vi "Render Non-Empty List Section.vi"(8 "Error In":errorcluster) -> (0 "Error Out":errorcluster)   [LabVIEW 2018, in "Tests.lvlib" / "Render.lvlib"]
uses:
  Render.lvlib
  <vilib>/addons/_JKI Toolkits/Caraya/classes/Test/Test.lvclass
  <vilib>/addons/_JKI Toolkits/Caraya/classes/Assert/Assert.lvclass
  src/Toolkit/Toolkit.lvlib
  src/Toolkit/Data/Map/Map.lvclass
  src/Toolkit/Data/Array/Array.lvclass
  src/Toolkit/Low-Level/Support/Lex String.vi
  src/Toolkit/Data/Map/Support/From Datum.vi
  src/Toolkit/Low-Level/Support/Render to String.vi
  src/Toolkit/Data/Array/Support/From Mapped Strings.vi
  src/Toolkit/Low-Level/Context/Compiler.lvclass
  D:/Users/cfield/Code/Field R&D Services/Labstache/src/Toolkit/Data/Datum/Datum.lvclass
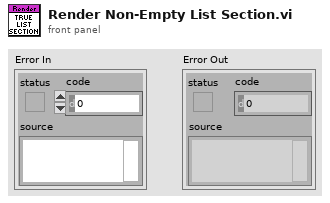
[diagram p1: front panel]
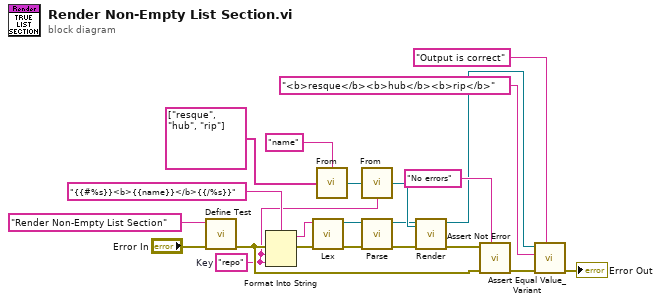
[diagram p0: block diagram]
diagram:
  w4 = "repo"  # Key
  n1 = call <vilib>:"Define Test.vi"("error in (no error)"="Error In", "Label (VI Title)"="Render Non-Empty List Section") -> ("error out"=w10:errorcluster)  [unwired: 9 in]
  n2 = Format Into String(format string="{{#%s}}<b>{{name}}</b>{{/%s}}", error in=w10, w4, w4) -> (resulting string=w7:string, error out=w9:errorcluster)  [unwired: 1 in]
  n3 = call-poly "Lex.vi"("Error In"=w9, "Context In"=w7) -> ("Error Out"=w12:errorcluster, "Context Out"=w13:refnum<class "Compiler.lvclass">)  [unwired: 7 in, 1 out]
  n4 = call-poly "From.vi"("Strings"=string[] ["resque", "hub", "rip"], "Key"="name") -> ("Array"=w5:refnum<class "Array.lvclass">)
  n5 = call-poly "From.vi"("Value"=w5, "Key"=w4) -> ("Map"=w11:refnum<class "Map.lvclass">)
  n6 = call "Parse.vi"("Error In"=w12, "Context In"=w13) -> ("Error Out"=w14:errorcluster, "Context Out"=w6:refnum<class "Compiler.lvclass">)  [unwired: 7 in, 1 out]
  n7 = call-poly "Render.vi"(7:w11, "Error In"=w14, "Context In"=w6) -> ("Error Out"=w16:errorcluster, "Context Out"=w15:refnum<class "Compiler.lvclass">)  [unwired: 6 in, 1 out]
  n8 = call <vilib>:"Assert Not Error.vi"("Label"="No errors", "error in (no error)"=w10, "Not Error?"=w16) -> ("error out"=w19:errorcluster)  [unwired: 8 in]
  n9 = call <vilib>:"Assert Equal Value_Variant.vi"("Label"="Output is correct", "error in (no error)"=w19, "Y"="<b>resque</b><b>hub</b><b>rip</b>", "X"=w15) -> ("error out"=→"Error Out":errorcluster)  [unwired: 7 in]
